vi "led.vi"() -> ()   [LabVIEW 2014]
panel:
  out "led":bool
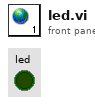
[diagram p1: front panel]
diagram:
